vi "3.5.vi"() -> ()   [LabVIEW 2017]
panel:
  out "数值 2":dbl
  in  "数值":dbl
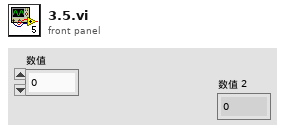
[diagram p1: front panel]
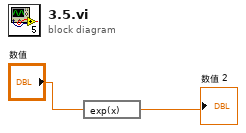
[diagram p0: block diagram]
diagram:
  n1 = expression code="exp(x)"("数值") -> (→"数值 2":dbl)
